vi "run.vi"(8 "error in (no error)":errorcluster, 11 "SAL_Listener in":refnum<class "SAL_Listener.lvclass">) -> (0 "error out":errorcluster, 3 "SAL_Listener out":refnum<class "SAL_Listener.lvclass">)   [LabVIEW 2016, in "SAL_Listener.lvclass"]
uses:
  SAL_Listener.lvclass
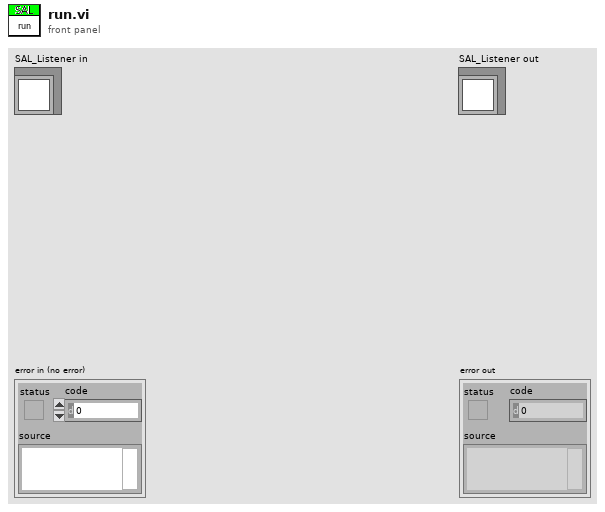
[diagram p1: front panel]
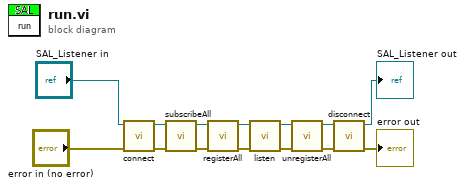
[diagram p0: block diagram]
diagram:
  n1 = call "connect.vi"("error in (no error)"="error in (no error)", "SAL_Listener in"="SAL_Listener in") -> ("error out"=w10:errorcluster, "SAL_Listener out"=w9:refnum<class "SAL_Listener.lvclass">)  [unwired: 8 in]
  n2 = call "subscribeAll.vi"("error in (no error)"=w10, "SAL_Listener in"=w9) -> ("error out"=w7:errorcluster, "SAL_Listener out"=w8:refnum<class "SAL_Listener.lvclass">)  [unwired: 8 in]
  n3 = call "registerAll.vi"("error in (no error)"=w7, "SAL_Listener in"=w8) -> ("error out"=w3:errorcluster, "SAL_Listener out"=w4:refnum<class "SAL_Listener.lvclass">)  [unwired: 8 in]
  n4 = call "listen.vi"("error in (no error)"=w3, "SAL_Listener in"=w4) -> ("error out"=w2:errorcluster, "SAL_Listener out"=w1:refnum<class "SAL_Listener.lvclass">)  [unwired: 8 in]
  n5 = call "unregisterAll.vi"("error in (no error)"=w2, "SAL_Listener in"=w1) -> ("error out"=w5:errorcluster, "SAL_Listener out"=w6:refnum<class "SAL_Listener.lvclass">)  [unwired: 8 in]
  n6 = call "disconnect.vi"("error in (no error)"=w5, "SAL_Listener in"=w6) -> ("error out"=→"error out":errorcluster, "SAL_Listener out"=→"SAL_Listener out":refnum<class "SAL_Listener.lvclass">)  [unwired: 8 in]
